vi "Git_ProgressWindow.vi"() -> ()   [LabVIEW 2012]
panel:
  in  "Cancel":bool
  in  "Message":string="Checking for updates, please wait."
  in  "Progress":u8(slide) scale=0.0..100.0
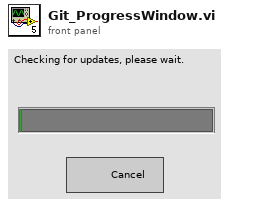
[diagram p1: front panel]
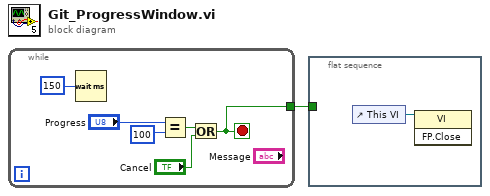
[diagram p0: block diagram]
diagram:
  n1 = while {
    tunnel: [w2] -> w1
    stop <- w2 stop-if-true
    n2 = Wait (ms)(milliseconds to wait=u32 150) -> ()  [unwired: 1 out]
    n3 = Equal?(x="Progress", y=u8 100) -> (x = y?=w5:bool)
    n4 = Or(x=w5, y="Cancel") -> (x .or. y?=w2:bool)
  }
  n5 = flat-sequence {
    tunnel: w1 -> [_]
    frame #0 {
      n6 = control-ref of="This VI"() -> (w8:refnum<vi>)
      n7 = invoke class="VI" method="FP.Close"(reference=w8) -> ()  [unwired: 2 in, 3 out]
    }
  }
